vi "Create.vi"   [LabVIEW 2018, in "Toolkit.lvlib" / "Known Hosts.lvclass"]
doc: "Creates a new Known Hosts objects and allocates memory within the libssh2lv shared library for a Known Hosts struct, which represents a linked list of known hosts."
uses:
  Known Hosts.lvclass
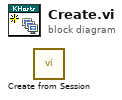
[diagram p0: block diagram]
diagram:
  n1 = call "Create from Session.vi"() -> ()  [unwired: 10 in, 2 out]
